vi "UDP Read.vi"(8 "error in (no error)":errorcluster, 11 "HPS17000 Refs in":refnum<class "HPS-17000.lvclass">[](array[class])) -> (0 "error out":errorcluster, 1 "last timestamp":i64, 2 "measurement array":T1[](array[typedef]), 3 "HPS17000 Refs out":refnum<class "HPS-17000.lvclass">[](array[class]))   [LabVIEW 2023, in "HPS-17000-PowerModule.lvlib" / "HPS-17000-PowerModule.lvclass"]
uses:
  HPS-17000-PowerModule.lvclass
  <instrlib>/HPS-17000/HPS-17000.lvclass
  builds/PowerModuleInterface/PowerModuleInterface.lvlibp/Classes/PowerModule_interface/Measurements.ctl
  HPS-17000-PowerModule.lvclass/HPS-17000-PowerModule.ctl
  <instrlib>/HPS-17000/Internal/Read Measurement Stream Multi.vi
  builds/PowerModuleInterface/PowerModuleInterface.lvlibp/Classes/PowerModule_interface/PowerModuleInterface.lvclass
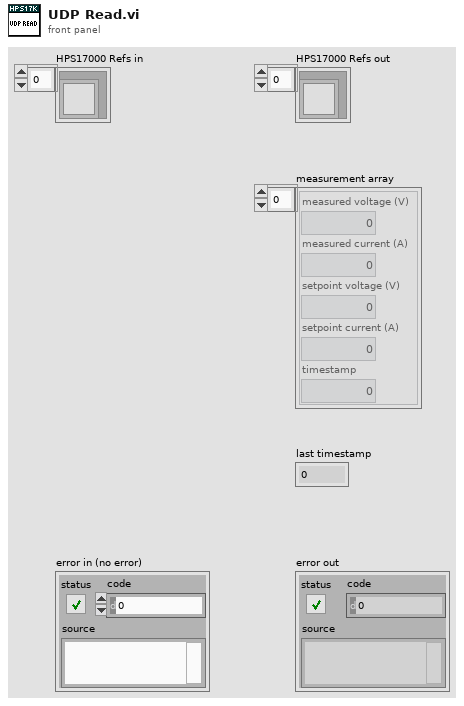
[diagram p1: front panel]
types:
  T1 = typedef "PowerModuleInterface.lvlibp/PowerModuleInterface.lvclass/Measurements.ctl" = cluster{"measured voltage (V)":dbl, "measured current (A)":dbl, "setpoint voltage (V)":dbl, "setpoint current (A)":dbl, "timestamp":dbl}
  T2 = typedef "NI_BC_client.lvlib/MStream_grpc_CyclerMeasurement.ctl" = cluster{"measured_voltage":sgl, "measured_current":sgl, "setpoint_voltage":sgl, "setpoint_current":sgl, "timestamp":i64}
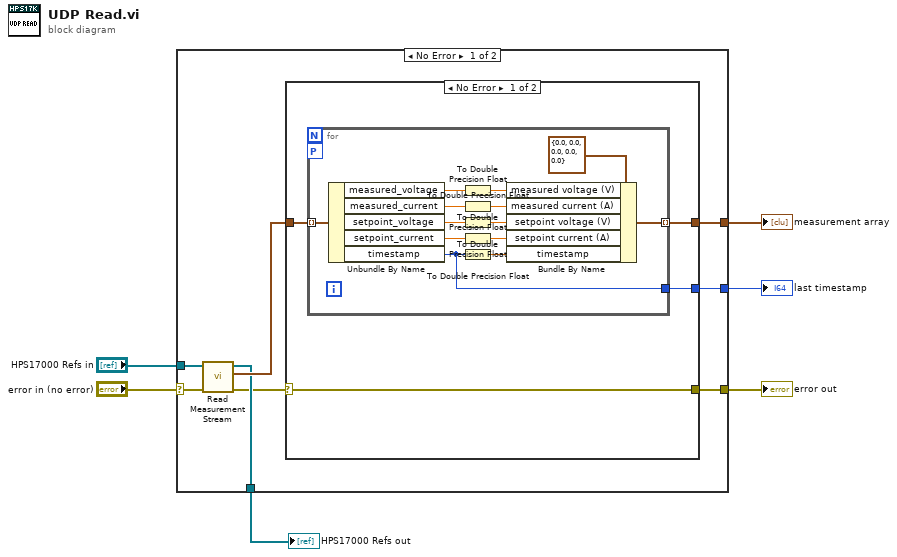
[diagram p0: block diagram]
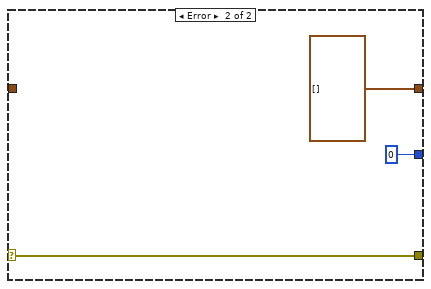
[diagram p2: hidden frame]
diagram:
  n1 = case shown="No Error" "error in (no error)" {
    selector: "error in (no error)" -> [w7 w35]
    tunnel: "HPS17000 Refs in" -> [w14 w36]
    tunnel: [w13 _] -> w5
    tunnel: [w12 _] -> w4
    tunnel: [w10 w36] -> w3
    tunnel: [w8 w35] -> w2
    frame No Error {
      n2 = call-poly <instrlib>:"Read Measurement Stream.vi"("error in"=w7, "cycler refs in"=w14) -> ("error out"=w9:errorcluster, "cycler measurements"=w11:T2[], "cycler refs out"=w10:refnum<class "HPS-17000.lvclass">[])  [unwired: 7 in]
      n3 = case shown="No Error" w9 {
        selector: w9 -> [w15 w32]
        tunnel: [w18 i64 0 ("timestamp")] -> w13
        tunnel: [w17 T1[] []] -> w12
        tunnel: w11 -> [w16 _]
        tunnel: [w15 w32] -> w8
        frame No Error {
          n4 = for {
            tunnel: w16 -> [w31] mode=indexing
            tunnel: [w22] -> w17 mode=indexing
            tunnel: [w20] -> w18
            workers-P: _ -> [_]
            n5 = Unbundle By Name(w31) -> ("measured_voltage"=w28:sgl, "measured_current"=w30:sgl, "setpoint_voltage"=w29:sgl, "setpoint_current"=w27:sgl, "timestamp"=w20:i64)
            n6 = To Double Precision Float(number=w28) -> (double precision float=w26:dbl)
            n7 = To Double Precision Float(number=w30) -> (double precision float=w25:dbl)
            n8 = To Double Precision Float(number=w29) -> (double precision float=w24:dbl)
            n9 = To Double Precision Float(number=w27) -> (double precision float=w23:dbl)
            n10 = To Double Precision Float(number=w20) -> (double precision float=w19:dbl)
            n11 = Bundle By Name(cluster=T1 {"measured voltage (V)"=0.0, "measured current (A)"=0.0, "setpoint voltage (V)"=0.0, "setpoint current (A)"=0.0, "timestamp"=0.0} ("Measurements"), "measured voltage (V)"=w26, "measured current (A)"=w25, "setpoint voltage (V)"=w24, "setpoint current (A)"=w23, "timestamp"=w19) -> (w22:T1)
          }
        }
        frame Error {
        }
      }
    }
    frame Error {
    }
  }
  "last timestamp" <- w5
  "measurement array" <- w4
  "HPS17000 Refs out" <- w3
  "error out" <- w2
